vi "udp_demonstration.vi"() -> ()   [LabVIEW 2018]
panel:
  in  "stop":bool
  out "data out":string
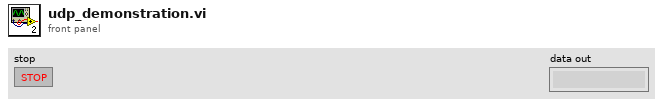
[diagram p1: front panel]
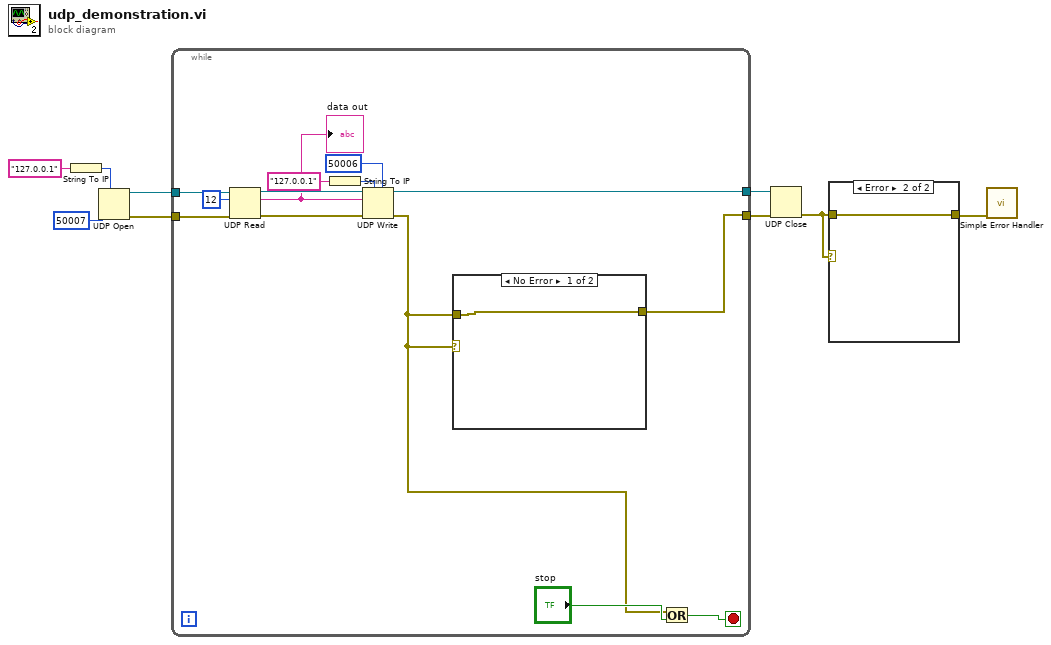
[diagram p0: block diagram]
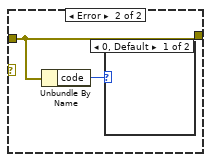
[diagram p3: hidden frame]
diagram:
  n1 = String To IP(1:"127.0.0.1" ("name")) -> (0:w2:u32)
  n2 = UDP Open(7:w2, 11:u16 50007 ("port")) -> (port=w9:refnum<k16>, 0:w8:errorcluster)  [unwired: 3 in, 1 out]
  n3 = while {
    tunnel: w9 -> [w22]
    tunnel: w8 -> [w23]
    tunnel: [w15] -> w7
    tunnel: [w14] -> w6
    stop <- w13 stop-if-true
    n4 = UDP Read(connection ID=w22, max size (548)=12, 8:w23) -> (data out=w10:string, error out=w20:errorcluster, 3:w19:refnum<k16>)  [unwired: 1 in, 2 out]
    "data out" <- w10
    n5 = String To IP(1:"127.0.0.1" ("name")) -> (0:w17:u32)
    n6 = UDP Write(address=w17, port or service name=u16 50006, connection ID=w19, data in=w10, 8:w20) -> (error out=w11:errorcluster, 3:w15:refnum<k16>)  [unwired: 1 in]
    n7 = case shown="No Error" w11 {
      tunnel: w11 -> [w24 w26]
      tunnel: [w24 w26] -> w14
      frame No Error {
      }
      frame Error {
        n8 = Unbundle By Name(w26) -> ("code"=w25:i32)
        n9 = case shown="0, Default" w25 {
          frame 0, Default {
          }
          frame 1 {
          }
        }
      }
    }
    n10 = Or(x=w11, y="stop") -> (x .or. y?=w13:bool)
  }
  n11 = UDP Close(connection ID=w7, 8:w6) -> (error out=w5:errorcluster)  [unwired: 1 out]
  n12 = case shown="Error" w5 {
    tunnel: [w27 w28] -> w4
    tunnel: w5 -> [w27 w28]
    frame No Error {
    }
    frame Error {
    }
  }
  n13 = call <vilib>:"Simple Error Handler.vi"("error in (no error)"=w4) -> ()  [unwired: 4 in, 5 out]
